vi "whilexample2.vi"() -> ()   [LabVIEW 2015]
panel:
  in  "stop":bool
  out "Es primo":bool
  in  "Ingrese un \nNumero\n(Entero)":i64
  out "Numero\n aleatorio":dbl
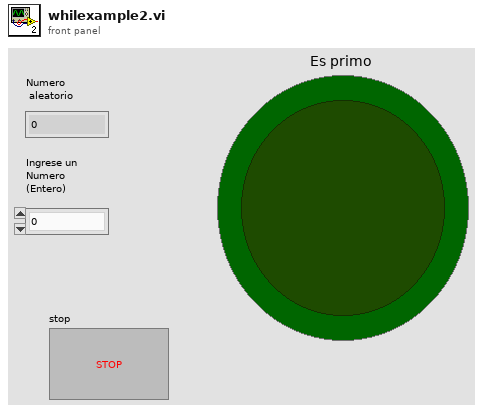
[diagram p1: front panel]
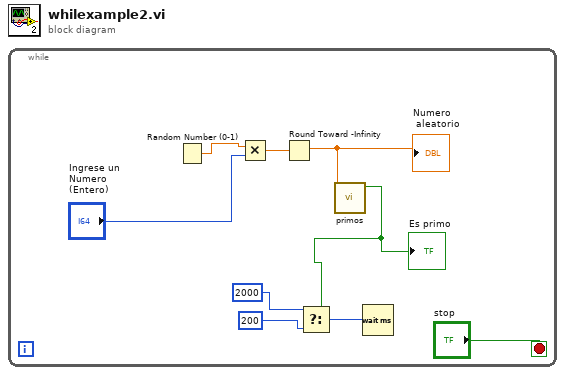
[diagram p0: block diagram]
diagram:
  n1 = while {
    stop <- "stop" stop-if-true
    n2 = Random Number (0-1)() -> (number: 0 to 1=w9:dbl)
    n3 = Multiply(x=w9, y="Ingrese un \nNumero\n(Entero)") -> (x*y=w8:dbl)
    n4 = Round Toward -Infinity(1:w8) -> (0:w6:dbl)
    "Numero\n aleatorio" <- w6
    n5 = call "primos.vi"("Numeric"=w6) -> ("Boolean"=w4:bool)  [unwired: 10 in]
    "Es primo" <- w4
    n6 = Select(t=2000, s=w4, f=u32 200 ("milliseconds to wait")) -> (s? t:f=w1:u32)
    n7 = Wait (ms)(milliseconds to wait=w1) -> ()  [unwired: 1 out]
  }
